vi "Asylum_SendIgorCommand.vi"(8 "error in (no error)":errorcluster, 9 "Format":string, 10 "command":string, 11 "Application":refnum<k7>) -> (0 "error out":errorcluster, 1 "history":string, 2 "results":string, 3 "Application":refnum<k7>)   [LabVIEW 2016]
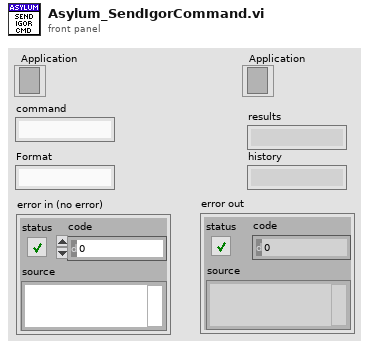
[diagram p1: front panel]
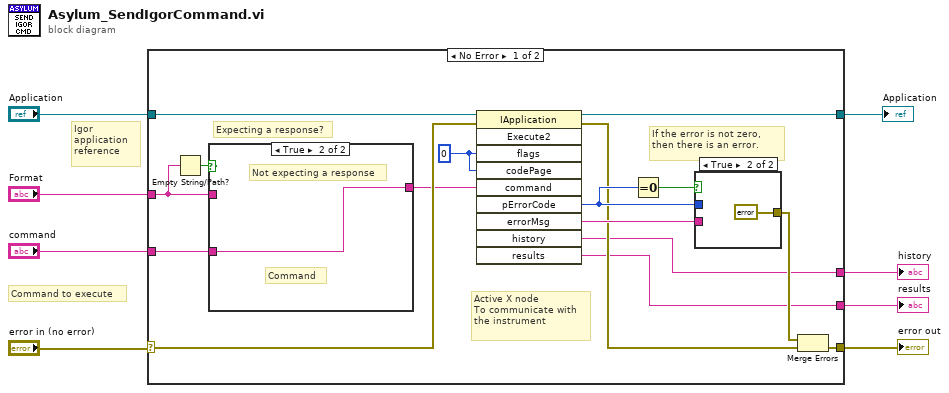
[diagram p0: block diagram]
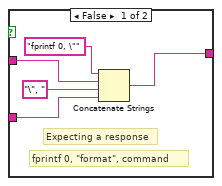
[diagram p2: hidden frame]
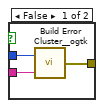
[diagram p3: hidden frame]
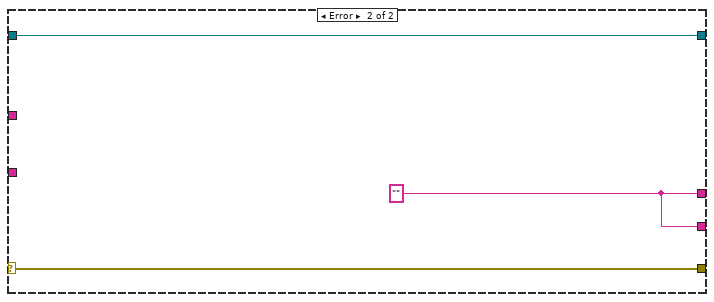
[diagram p4: hidden frame]
diagram:
  # "Command to execute"
  # "Igor application reference"
  n1 = case shown="No Error" "error in (no error)" {
    selector: "error in (no error)" -> [w23 w37]
    tunnel: [w16 w37] -> w8
    tunnel: "Application" -> [w24 w35]
    tunnel: "command" -> [w10 _]
    tunnel: [w15 w36] -> w4
    tunnel: [w14 w36] -> w3
    tunnel: [w13 w35] -> w2
    tunnel: "Format" -> [w9 _]
    frame No Error {
      w22 = 0 ("flags")
      # "Expecting a response?"
      # "Active X node\nTo communicate with the instrument"
      # "If the error is not zero, then there is an error."
      n2 = Empty String/Path?(string/path=w9) -> (empty?=w12:bool)
      n3 = case shown="True" w12 {
        tunnel: [w25 w30] -> w11
        tunnel: w10 -> [w26 w30]
        tunnel: w9 -> [w28 _]
        frame False {
          # "Expecting a response"
          # "fprintf 0, \"format\", command"
          n4 = Concatenate Strings("fprintf 0, \"" ("string"), w28, "\", " ("string"), w26) -> (w25:string)
        }
        frame True {
          # "Not expecting a response"
          # "Command"
        }
      }
      n5 = invoke class="IApplication" method="Execute2"(reference=w24, error in=w23, "flags"=w22, "codePage"=w22, "command"=w11) -> (reference out=w13:refnum<k7>, error out=w17:errorcluster, "pErrorCode"=w20:i32, "errorMsg"=w19:string, "history"=w15:string, "results"=w14:string)  [unwired: 5 in, 4 out]
      n6 = Equal To 0?(x=w20) -> (x = 0?=w21:bool)
      n7 = case shown="True" w21 {
        tunnel: w20 -> [w33 _]
        tunnel: w19 -> [w32 _]
        tunnel: [w31 errorcluster {"status"=FALSE, "code"=0, "source"=""} ("error constant")] -> w18
        frame False {
          n8 = call <userlib>:"Build Error Cluster__ogtk.vi"("String to Prepend to source (\"\")"=w32, "code"=w33) -> ("error out"=w31:errorcluster)
        }
        frame True {
        }
      }
      n9 = Merge Errors(w18, w17) -> (w16:errorcluster)
    }
    frame Error {
      w36 = "" ("history")
    }
  }
  "error out" <- w8
  "history" <- w4
  "results" <- w3
  "Application" <- w2
